vi "Build-timeline.vi"(8 "error in (no error)":errorcluster, 10 "Temp-timeline in":T1, 11 "Attribute in":refnum<class "LaserPowerDelay.lvclass">) -> (0 "error out":errorcluster, 2 "Temp-timeline":T1, 3 "Attribute out":refnum<class "LaserPowerDelay.lvclass">)   [LabVIEW 2013, in "MaterialCharacterization.lvlib" / "LaserPowerDelay.lvclass"]
uses:
  LaserPowerDelay.lvclass
  ScanParser/Path-buffer.ctl
  ScanParser/Point-buffer.ctl
  Element-XML/Elements.ctl
  ScanParser/Property-buffer.ctl
  ScanParser/Units.ctl
  ScanParser/Speed.ctl
  Time/Time.lvclass/Time.ctl
  Time/Read Time interval.vi
  Element-XML/Element-XML.lvclass
  ScanParser/MC-ScanParser.lvclass
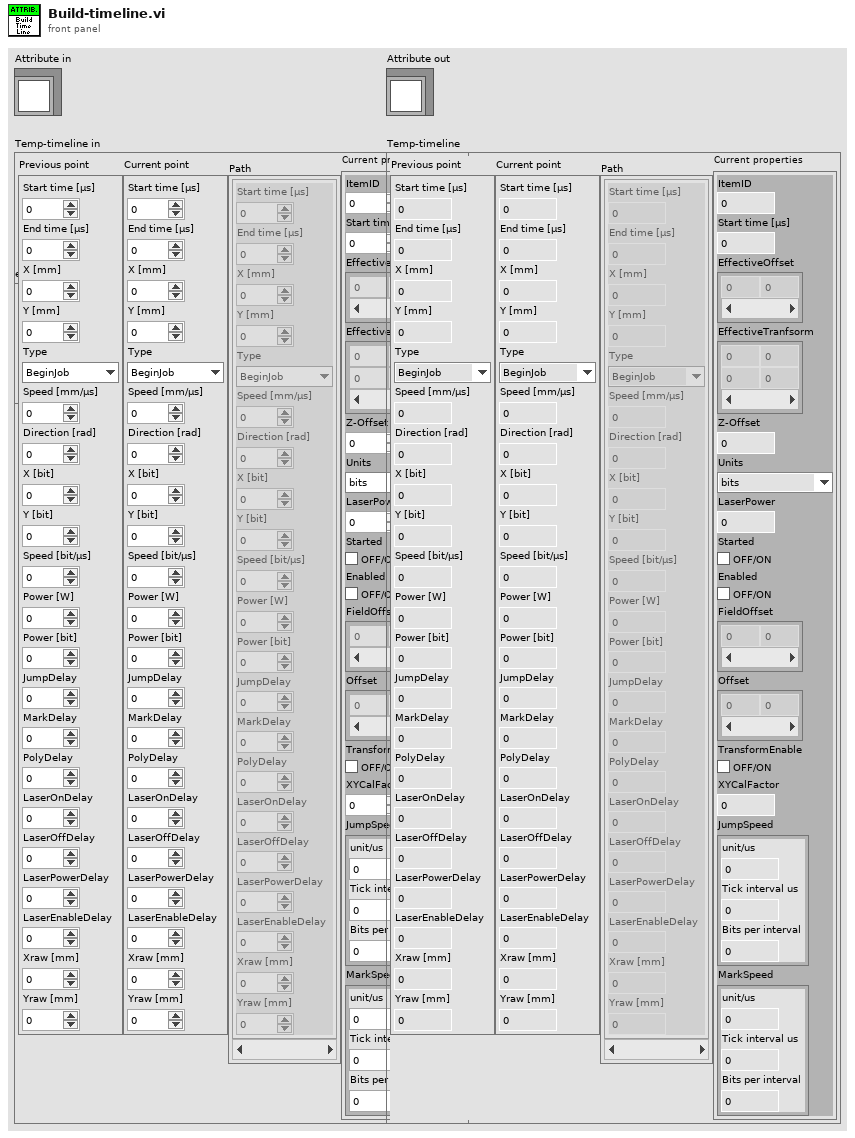
[diagram p1: front panel]
types:
  T1 = typedef "MaterialCharacterization.lvlib/MC-ScanParser.lvclass/Path-buffer.ctl" = cluster{"Previous point":T2, "Current point":T2, "Path":T2[], "Current properties":T4}
  T2 = typedef "MaterialCharacterization.lvlib/MC-ScanParser.lvclass/Point-buffer.ctl" = cluster{"Start time [µs]":i64, "End time [µs]":i64, "X [mm]":dbl, "Y [mm]":dbl, "Type":T3, "Speed [mm/µs]":dbl, "Direction [rad]":dbl, "X [bit]":i16, "Y [bit]":i16, "Speed [bit/µs]":dbl, "Power [W]":dbl, "Power [bit]":u8, "JumpDelay":i64, "MarkDelay":i64, "PolyDelay":i64, "LaserOnDelay":i64, "LaserOffDelay":i64, "LaserPowerDelay":i64, "LaserEnableDelay":i64, "Xraw [mm]":dbl, "Yraw [mm]":dbl}
  T3 = typedef "MaterialCharacterization.lvlib/Element-XML.lvclass/Elements.ctl" = enum16{"BeginJob", "WriteDigital", "WriteAnalog", "Set", "ApplicationEvent", "JumpAbs", "MarkAbs", "JumpRel", "MarkRel", "LongDelay", "EndJob"}
  T4 = typedef "MaterialCharacterization.lvlib/MC-ScanParser.lvclass/Property-buffer.ctl" = cluster{"ItemID":u32, "Start time":i64, "EffectiveOffset":dbl[], "EffectiveTranfsorm":dbl[][], "Z-Offset":sgl, "Units":T5, "LaserPower":u8, "Started":bool, "Enabled":bool, "FieldOffset":dbl[], "Offset":dbl[], "TransformEnable":bool, "XYCalFactor":dbl, "JumpSpeed":T6, "MarkSpeed":T6}
  T5 = typedef "MaterialCharacterization.lvlib/MC-ScanParser.lvclass/Units.ctl" = enum16{"bits", "mm", "inch", "mils"}
  T6 = typedef "MaterialCharacterization.lvlib/MC-ScanParser.lvclass/Speed.ctl" = cluster{"unit/us":dbl, "Tick interval us":u16, "Bits per interval":u16}
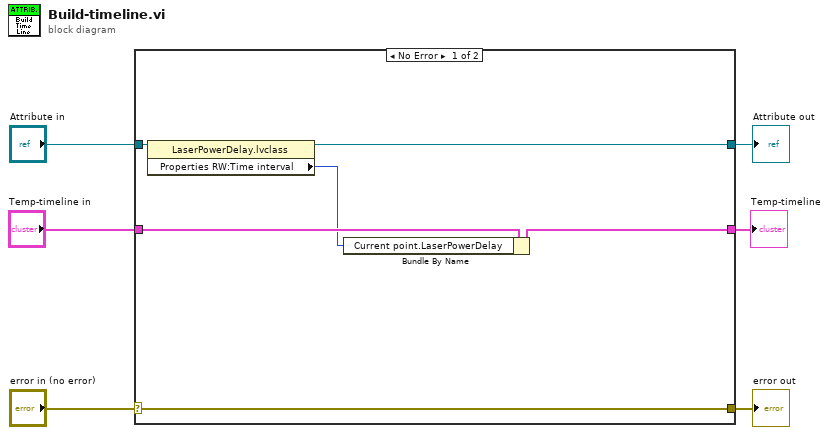
[diagram p0: block diagram]
diagram:
  n1 = case shown="No Error" "error in (no error)" {
    selector: "error in (no error)" -> [w9 w15]
    tunnel: [w9 w15] -> w5
    tunnel: [w11 w14] -> w3
    tunnel: "Attribute in" -> [w12 w14]
    tunnel: "Temp-timeline in" -> [w10 w13]
    tunnel: [w8 w13] -> w1
    frame No Error {
      n2 = property class="LaserPowerDelay.lvclass"(reference=w12) -> (reference out=w11:refnum<class "LaserPowerDelay.lvclass">, "Properties RW:Time interval"=w7:i64)  [unwired: 1 in, 1 out]
      n3 = Bundle By Name(cluster=w10, "Current point.LaserPowerDelay"=w7) -> (w8:T1)
    }
    frame Error {
    }
  }
  "error out" <- w5
  "Attribute out" <- w3
  "Temp-timeline" <- w1
